vi "Inverter Status.vi"(0 "GEA2 Reference In":refnum<k24>, 1 "GEA Inputs":T3={"Source"=228, "Destination"=35} {"Destination" format="%.0x"; "Source" format="%.0x"}, 2 "Standalone?":bool, 5 "Error In":errorcluster) -> (14 "GEA2 Reference Out":refnum<k24>, 15 "Inverter Command Status":T1={"Command State"="Unknown State", "Command ID"="Dry Load Sense", "Command Sequence #"=0}, 16 "Inverter Status Out":T2, 19 "Error Out":errorcluster)   [LabVIEW 2016]
uses:
  Q:/Common/DLLs/GEA3/GeaCommunication.dll
  Common/DLLs/GEA3/GeaCommunication.dll
  Common/LabVIEW GEA2 Toolkit/LabVIEW_GEA2_Toolkit.lvlibp/type defs/Source_Destination.ctl
  Type Defs/CommandStatus.ctl
  Common/LabVIEW GEA2 Toolkit/LabVIEW_GEA2_Toolkit.lvlibp/type defs/ERD Read Data In.ctl
  Common/LabVIEW GEA2 Toolkit/LabVIEW_GEA2_Toolkit.lvlibp/type defs/Data Type.ctl
  Common/LabVIEW GEA2 Toolkit/LabVIEW_GEA2_Toolkit.lvlibp
panel:
  in  "Inverter Status":T2={"Inverter Cmd Status"={"Command State"="Unknown State", "Command ID"="Dry Load Sense", "Command Sequence #"=0}, "Requested Power Level"="Full", "Actual Power Level"="", "Command Status"="Fault", "Command Request"="", "Inverter Heartbeat"=FALSE}
  in  "Inverter Cmd Status Control":T1={"Command State"="Unknown State", "Command ID"="Dry Load Sense", "Command Sequence #"=0}
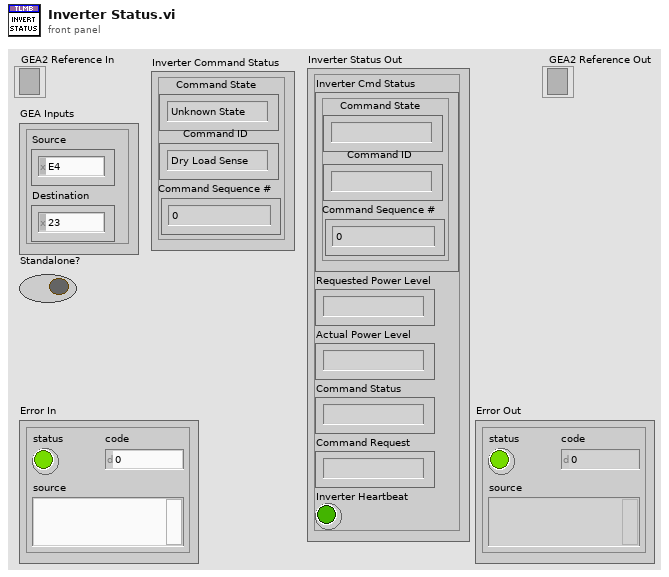
[diagram p1: front panel]
types:
  T1 = typedef "CommandStatus.ctl" = cluster{"Command State":string, "Command ID":string, "Command Sequence #":u32}
  T2 = cluster{"Inverter Cmd Status":T1, "Requested Power Level":string, "Actual Power Level":string, "Command Status":string, "Command Request":string, "Inverter Heartbeat":bool}
  T3 = typedef "LabVIEW_GEA2_Toolkit.lvlibp/Source_Destination.ctl" = cluster{"Source":u8, "Destination":u8}
  T4 = typedef "LabVIEW_GEA2_Toolkit.lvlibp/ERD Read Data In.ctl" = cluster{"ERD Number":u16, "Data Type":T5}
  T5 = typedef "LabVIEW_GEA2_Toolkit.lvlibp/Data Type.ctl" = enum16{"string", "boolean", "uint8_t", "uint16_t", "uint32_t", "uint64_t", "int8_t", "int16_t", "int32_t", "int64_t"}
  T6 = typedef "LabVIEW_GEA2_Toolkit.lvlibp/ERD Read Data Out.ctl" = cluster{"ERD Number":u16, "Data":string}
  T7 = cluster{"ERD Data Out[0]":T6, "ERD Data Out[1]":T6, "ERD Data Out[2]":T6, "ERD Data Out[3]":T6, "ERD Data Out[4]":T6, "ERD Data Out[5]":T6, "ERD Data Out[6]":T6, "ERD Data Out[7]":T6, "ERD Data Out[8]":T6}
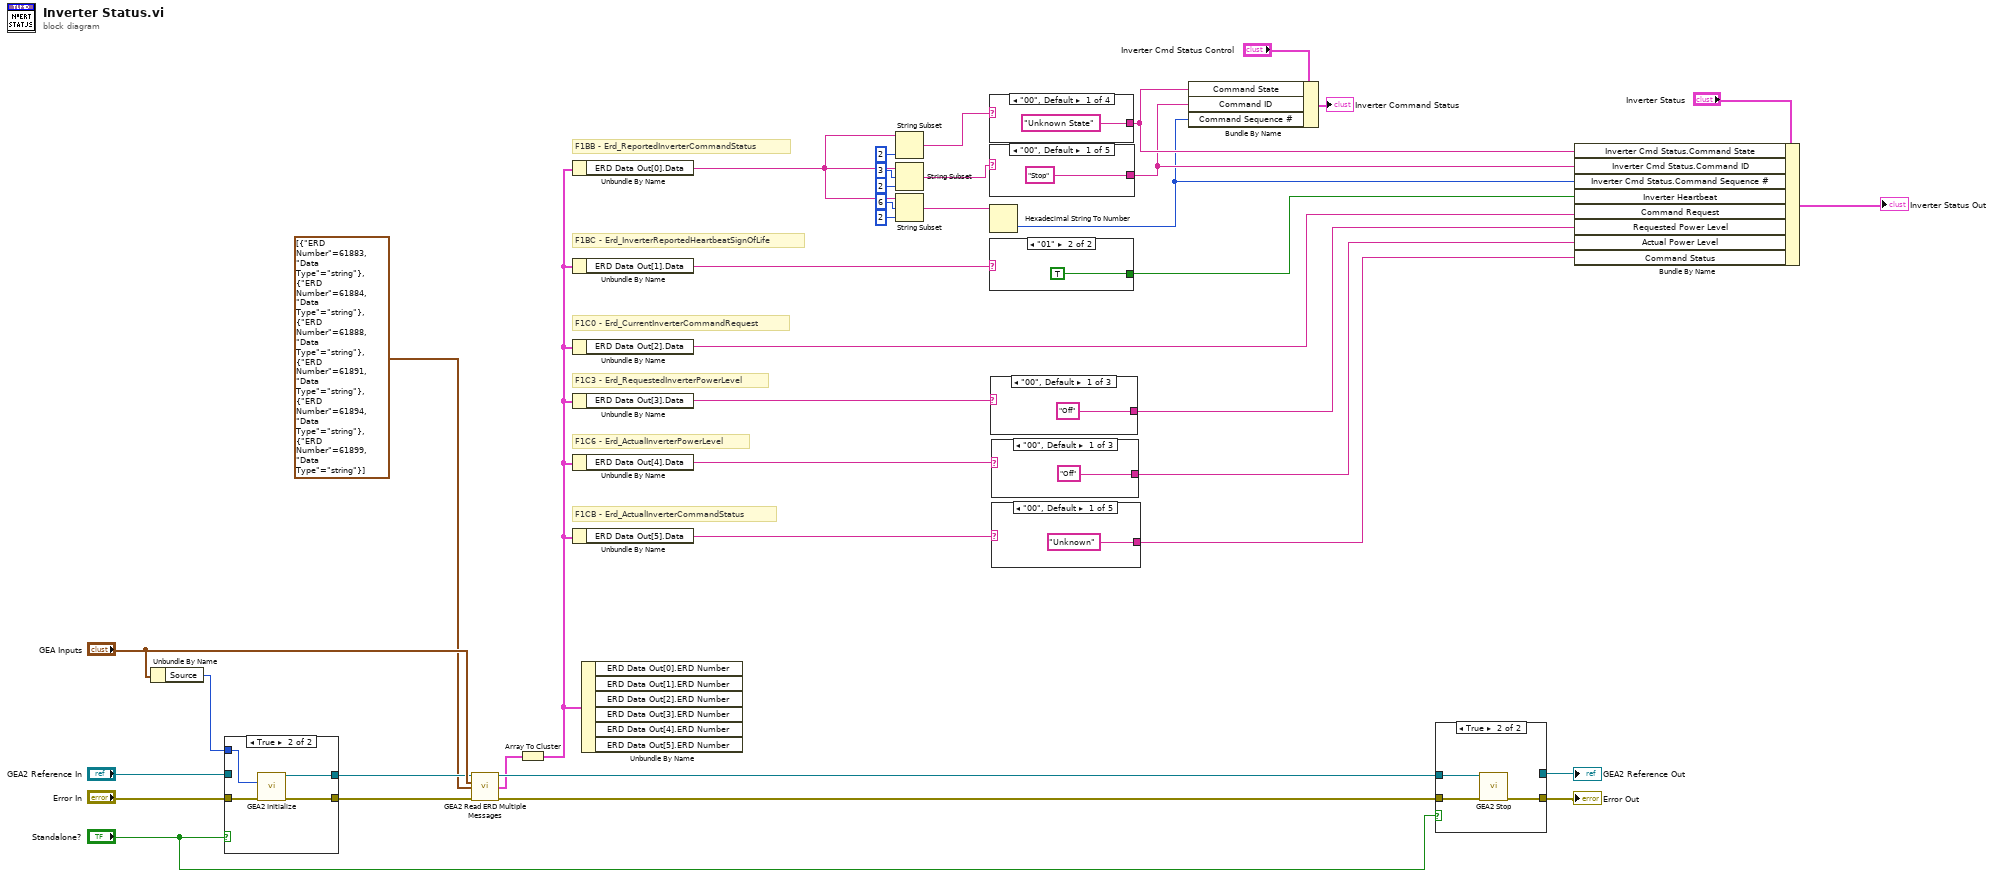
[diagram p0: block diagram]
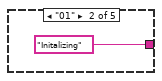
[diagram p2: hidden frame]
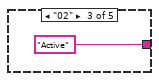
[diagram p3: hidden frame]
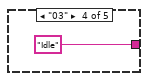
[diagram p4: hidden frame]
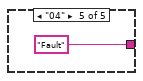
[diagram p5: hidden frame]
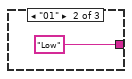
[diagram p6: hidden frame]
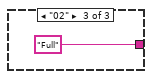
[diagram p7: hidden frame]
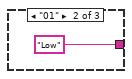
[diagram p8: hidden frame]
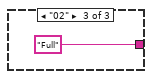
[diagram p9: hidden frame]
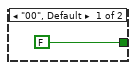
[diagram p10: hidden frame]
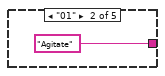
[diagram p11: hidden frame]
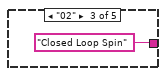
[diagram p12: hidden frame]
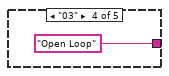
[diagram p13: hidden frame]
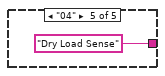
[diagram p14: hidden frame]
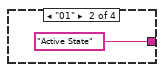
[diagram p15: hidden frame]
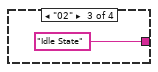
[diagram p16: hidden frame]
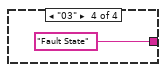
[diagram p17: hidden frame]
diagram:
  # "F1CB - Erd_ActualInverterCommandStatus"
  # "F1C6 - Erd_ActualInverterPowerLevel"
  # "F1C3 - Erd_RequestedInverterPowerLevel"
  # "F1C0 - Erd_CurrentInverterCommandRequest"
  # "F1BC - Erd_InverterReportedHeartbeatSignOfLife"
  # "F1BB - Erd_ReportedInverterCommandStatus"
  n1 = Unbundle By Name("GEA Inputs") -> ("Source"=w39:u8)
  n2 = case shown="True" "Standalone?" {
    tunnel: w39 -> [_ w45]
    tunnel: "Error In" -> [w40 w44]
    tunnel: "GEA2 Reference In" -> [w41 _]
    tunnel: [w41 w43] -> w35
    tunnel: [w40 w42] -> w34
    frame False {
    }
    frame True {
      n3 = call "GEA2 Initialize.vi"("Source Address"=w45, "error in"=w44) -> ("GEA2 Reference Out"=w43:refnum<k24>, "error out"=w42:errorcluster)  [unwired: 11 in, 1 out]
    }
  }
  n4 = call "GEA2 Read ERD Multiple Messages.vi"("GEA2 Reference In"=w35, "GEA Inputs"="GEA Inputs", "Read ERD List"=T4[] [{"ERD Number"=61883, "Data Type"=enum."string"}, {"ERD Number"=61884, "Data Type"=enum."string"}, {"ERD Number"=61888, "Data Type"=enum."string"}, {"ERD Number"=61891, "Data Type"=enum."string"}, {"ERD Number"=61894, "Data Type"=enum."string"}, {"ERD Number"=61899, "Data Type"=enum."string"}], "Error In"=w34) -> ("GEA2 Reference Out"=w33:refnum<k24>, "ERD Data Out"=w28:T6[], "Error Out"=w32:errorcluster)  [unwired: 8 in, 1 out]
  n5 = Array To Cluster(array=w28) -> (cluster=w17:T7)
  n6 = Unbundle By Name(w17) -> ("ERD Data Out[0].Data"=w22:string)
  n7 = Unbundle By Name(w17) -> ("ERD Data Out[1].Data"=w16:string)
  n8 = Unbundle By Name(w17) -> ("ERD Data Out[2].Data"=w11:string)
  n9 = Unbundle By Name(w17) -> ("ERD Data Out[3].Data"=w15:string)
  n10 = Unbundle By Name(w17) -> ("ERD Data Out[4].Data"=w14:string)
  n11 = Unbundle By Name(w17) -> ("ERD Data Out[5].Data"=w13:string)
  n12 = Unbundle By Name(w17) -> ()  [unwired: 6 out]
  n13 = String Subset(string=w22, length (rest)=2 ("length (rest)")) -> (substring=w21:string)  [unwired: 1 in]
  n14 = String Subset(string=w22, offset (0)=3, length (rest)=2 ("length (rest)")) -> (substring=w20:string)
  n15 = String Subset(string=w22, offset (0)=6, length (rest)=2 ("length (rest)")) -> (substring=w19:string)
  n16 = case shown="\"00\", Default" w21 {
    tunnel: ["Unknown State" "Active State" "Idle State" "Fault State"] -> w5
    frame "00", Default {
    }
    frame "01" {
    }
    frame "02" {
    }
    frame "03" {
    }
  }
  n17 = case shown="\"00\", Default" w20 {
    tunnel: ["Stop" "Agitate" "Closed Loop Spin" "Open Loop" "Dry Load Sense"] -> w4
    frame "00", Default {
    }
    frame "01" {
    }
    frame "02" {
    }
    frame "03" {
    }
    frame "04" {
    }
  }
  n18 = Hexadecimal String To Number(string=w19) -> (number=w3:u32)  [unwired: 2 in, 1 out]
  n19 = case shown="\"01\"" w16 {
    tunnel: [FALSE TRUE] -> w12
    frame "00", Default {
    }
    frame "01" {
    }
  }
  n20 = case shown="\"00\", Default" w15 {
    tunnel: ["Off" "Low" "Full"] -> w10
    frame "00", Default {
    }
    frame "01" {
    }
    frame "02" {
    }
  }
  n21 = case shown="\"00\", Default" w14 {
    tunnel: ["Off" "Low" "Full"] -> w9
    frame "00", Default {
    }
    frame "01" {
    }
    frame "02" {
    }
  }
  n22 = case shown="\"00\", Default" w13 {
    tunnel: ["Unknown" "Initalizing" "Active" "Idle" "Fault"] -> w8
    frame "00", Default {
    }
    frame "01" {
    }
    frame "02" {
    }
    frame "03" {
    }
    frame "04" {
    }
  }
  n23 = Bundle By Name(cluster="Inverter Cmd Status Control", "Command State"=w5, "Command ID"=w4, "Command Sequence #"=w3) -> (→"Inverter Command Status":T1)
  n24 = case shown="True" "Standalone?" {
    tunnel: w33 -> [w69 w72]
    tunnel: w32 -> [w68 w71]
    tunnel: [w69 _] -> w31
    tunnel: [w68 w70] -> w30
    frame False {
    }
    frame True {
      n25 = call "GEA2 Stop.vi"("GEA2 Reference In"=w72, "Error In"=w71) -> ("Error Out"=w70:errorcluster)  [unwired: 13 in]
    }
  }
  "GEA2 Reference Out" <- w31
  "Error Out" <- w30
  n26 = Bundle By Name(cluster="Inverter Status", "Inverter Cmd Status.Command State"=w5, "Inverter Cmd Status.Command ID"=w4, "Inverter Cmd Status.Command Sequence #"=w3, "Inverter Heartbeat"=w12, "Command Request"=w11, "Requested Power Level"=w10, "Actual Power Level"=w9, "Command Status"=w8) -> (→"Inverter Status Out":T2)
